vi "XY Graph Sum Selected Plots Event.vi"(8 "Error In":errorcluster, 9 "Add All Plots? (F)":bool, 11 "XYGraph Ref":T1) -> (0 "Error Out":errorcluster, 1 "Message":string, 2 "Sum Plot Name":string, 3 "Added Plot Names":string[](array[string]), 4 "Added Plot Indices":i32[](array[numeric]), 5 "Graph Name":string)   [LabVIEW 2021, in "XY Graph Add-Ons.lvlib"]
uses:
  XY Graph Add-Ons.lvlib
  XY Graph Refnum.ctl
  <userlib>/_OpenG.lib/array/array.llb/Index 1D Array Elements (Variant)__ogtk.vi
  XY Graph Add Single Plot with Name.vi
  <userlib>/_OpenG.lib/array/array.llb/openg_array.lvlib
  Strings/Strings.lvlib
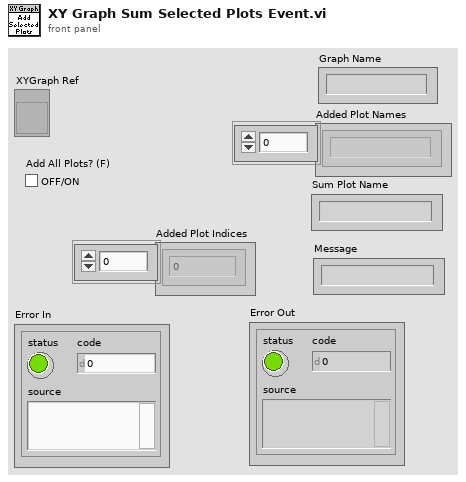
[diagram p1: front panel]
types:
  T1 = typedef "XY Graph Add-Ons.lvlib/XY Graph Refnum.ctl" = refnum<vi>
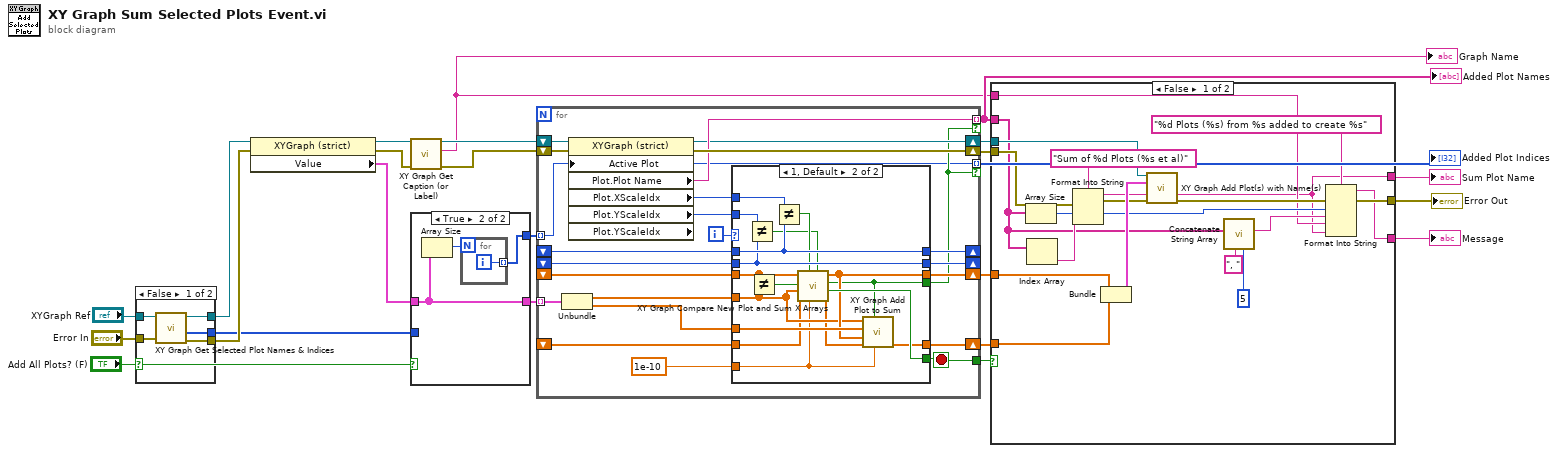
[diagram p0: block diagram]
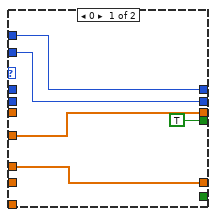
[diagram p3: hidden frame]
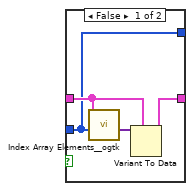
[diagram p4: hidden frame]
diagram:
  n1 = case shown="False" "Add All Plots? (F)" {
    tunnel: "XYGraph Ref" -> [w29 w31]
    tunnel: "Error In" -> [w28 w30]
    tunnel: [w27 w31] -> w22
    tunnel: [w26 _] -> w18
    tunnel: [w25 w30] -> w20
    frame False {
      n2 = call "XY Graph Get Selected Plot Names & Indices.vi"("error in (no error)"=w28, "XYGraph in"=w29) -> ("error out"=w25:errorcluster, "Selected Plots"=w26:i32[], "XYGraph out"=w27:T1)  [unwired: 5 in, 2 out]
    }
    frame True {
    }
  }
  n3 = property class="XYGraph (strict)"(reference=w22, error in=w20) -> (reference out=w5:T1, error out=w3:errorcluster, "Value"=w21:cluster{"X Array":dbl[], "Y Array":dbl[]}[])
  n4 = call "XY Graph Get Caption (or Label).vi"("error in (no error)"=w3, "XYGraph in"=w5) -> ("error out"=w2:errorcluster, "Caption (or Label) Text"=w1:string, "XYGraph out"=w4:T1)  [unwired: 7 in]
  "Graph Name" <- w1
  n5 = case shown="True" "Add All Plots? (F)" {
    tunnel: w21 -> [w34 w38]
    tunnel: [w33 w38] -> w17
    tunnel: w18 -> [w32 _]
    tunnel: [w32 w36] -> w8
    frame False {
      n6 = call-poly <userlib>:"Index Array Elements__ogtk.vi"("indices"=w32, "array"=w34) -> ("elements"=w35:variant[])  [unwired: 9 in]
      n7 = Variant To Data(type=w34, Variant=w35) -> (data=w33:cluster{"X Array":dbl[], "Y Array":dbl[]}[])  [unwired: 1 in, 1 out]
    }
    frame True {
      n8 = Array Size(array=w38) -> (size(s)=w37:i32)
      n9 = for {
        N: w37 -> [_]
        tunnel: [w39] -> w36 mode=indexing
        i -> [w39]
      }
    }
  }
  n10 = for {
    tunnel: w17 -> [w62] mode=indexing
    tunnel: [w58] -> w9 mode=indexing if=w43
    tunnel: [w40] -> w11 mode=indexing if=w43
    shift-right: [w55] -> _
    shift-left: _ -> [w50]
    shift-right: [w54] -> _
    shift-left: _ -> [w49]
    shift-right: [w51] -> w16
    shift-left: _ -> [w48]
    shift-right: [w46] -> w15
    shift-left: _ -> [w45]
    shift-right: [w59] -> w14
    shift-left: w2 -> [w60]
    shift-right: [w44] -> w12
    shift-left: w4 -> [w61]
    tunnel: [w42] -> w10
    tunnel: w8 -> [w40] mode=indexing
    i -> [w57]
    stop <- w42 stop-if-true
    n11 = Unbundle(w62) -> ("X Array"=w52:dbl[], "Y Array"=w47:dbl[])
    n12 = property class="XYGraph (strict)" props=["Active Plot", "Plot", "Plot Name", "Plot", "XScaleIdx", "Plot", "YScaleIdx", "Plot", "YScaleIdx"](reference=w61, error in=w60, "Active Plot"=w40) -> (reference out=w44:T1, error out=w59:errorcluster, "Plot.Plot Name"=w58:string, "Plot.XScaleIdx"=w56:u32, "Plot.YScaleIdx"=w53:u32)  [unwired: 1 out]
    n13 = case shown="1, Default" w57 {
      tunnel: w56 -> [w67 w84]
      tunnel: [w67 w83] -> w55
      tunnel: [w66 w81] -> w54
      tunnel: w53 -> [w66 w82]
      tunnel: [w65 w74] -> w51
      tunnel: w52 -> [w65 w71]
      tunnel: w50 -> [_ w83]
      tunnel: w49 -> [_ w81]
      tunnel: w48 -> [_ w77]
      tunnel: w47 -> [w64 w75]
      tunnel: [w64 w73] -> w46
      tunnel: w45 -> [_ w70]
      tunnel: [_ w76] -> w42
      tunnel: [TRUE w72] -> w43
      tunnel: 1e-10 ("epsilon (machine)") -> [_ w68]
      frame 0 {
      }
      frame 1, Default {
        n14 = Not Equal?(x=w82, y=w81) -> (x != y?=w79:bool)
        n15 = Not Equal?(x=w77, y=w71) -> (x != y?=w78:bool)
        n16 = Not Equal?(x=w84, y=w83) -> (x != y?=w80:bool)
        n17 = call "XY Graph Compare New Plot and Sum X Arrays.vi"("Different Y Scale"=w79, "epsilon (machine)"=w68, "Different X Scale"=w80, "Existing Y Array"=w70, "New X Array in"=w71, "Different X Axis"=w78, "Existing X Array"=w77) -> ("Y Array out"=w69:dbl[], "Cancel"=w76:bool, "Keep Plot"=w72:bool, "X Array out"=w74:dbl[])  [unwired: 1 in]
        n18 = call "XY Graph Add Plot to Sum.vi"("epsilon (machine)"=w68, "Keep Plot"=w72, "Sum Plot Y"=w69, "Sum Plot X"=w74, "New Plot Y"=w75, "New Plot X"=w71) -> ("Sum Plot Y"=w73:dbl[])  [unwired: 5 in]
      }
    }
  }
  "Added Plot Indices" <- w11
  "Added Plot Names" <- w9
  n19 = case shown="False" w10 {
    tunnel: w16 -> [w104 _]
    tunnel: w15 -> [w103 _]
    tunnel: w14 -> [w98 w105]
    tunnel: [w88 w105] -> w13
    tunnel: [w85 _] -> w7
    tunnel: w12 -> [w101 _]
    tunnel: w9 -> [w92 _]
    tunnel: [w87 _] -> w6
    tunnel: w1 -> [w86 _]
    frame False {
      n20 = Array Size(array=w92) -> (size(s)=w91:i32)
      n21 = Index Array(array=w92) -> (element=w96:string)  [unwired: 1 in]
      n22 = Format Into String(format string="Sum of %d Plots (%s et al)" ("initial string"), error in=w98, w91, w96) -> (resulting string=w100:string, error out=w99:errorcluster)  [unwired: 1 in]
      n23 = Bundle("X Array out"=w104, "Sum Plot Y"=w103) -> (w102:cluster{"X Array out":dbl[], "Sum Plot Y":dbl[]})  [unwired: 1 in]
      n24 = call-poly "XY Graph Add Plot(s) with Name(s).vi"("XYGraph Ref in"=w101, "Plot"=w102, "Plot Name (\"Plot\")"=w100, "error in (no error)"=w99) -> ("Plot Name"=w85:string, "error out"=w89:errorcluster)  [unwired: 8 in, 2 out]
      n25 = call "Concatenate String Array.vi"("Max Number of Elements (None: -1)"=5 ("Max Number of Elements (None: 1)"), "Separator (TAB)"=", ", "String Array"=w92) -> ("Formatted String"=w94:string)  [unwired: 8 in]
      n26 = Format Into String(format string="%d Plots (%s) from %s added to create %s", error in=w89, w91, w94, w86, w85) -> (resulting string=w87:string, error out=w88:errorcluster)  [unwired: 1 in]
    }
    frame True {
    }
  }
  "Error Out" <- w13
  "Message" <- w6
  "Sum Plot Name" <- w7
